vi "PhotonPoseEstimator_EstimatePnpDistanceTrigSolvePose.vi"(10 "CameraResult":T15={"Targets"=[], "PhotonMultiTargetPNPResult"={"PhotonPNPResult"={"IsPresent"=FALSE, "bestReprojErr"=0.0, "altReprojErr"=0.0, "ambiguity"=0.0, "Best"={"TRANSLATION3D"={"X"=0.0, "Y"=0.0, "Z"=0.0}, "ROTATION3D"={"Q_quaternion"={"R"=1.0, "V"=[0.0, 0.0, 0.0]}}, "XF"=FALSE}, "Alt"={"TRANSLATION3D"={"X"=0.0, "Y"=0.0, "Z"=0.0}, "ROTATION3D"={"Q_quaternion"={"R"=1.0, "V"=[0.0, 0.0, 0.0]}}, "XF"=FALSE}}, "FiducialIDsUsed"=[]}, "PhotonPipelineMetadata"={"CaptureTimestampMicros"=0, "PublishTimestampMicros"=0, "SequenceID"=0, "TimeSinceLastPong"=0}} {"PhotonMultiTargetPNPResult"."PhotonPNPResult"."Alt"."TRANSLATION3D"."Z" format="%14.3f"; "PhotonMultiTargetPNPResult"."PhotonPNPResult"."Alt"."TRANSLATION3D"."Y" format="%14.3f"; "PhotonMultiTargetPNPResult"."PhotonPNPResult"."Alt"."TRANSLATION3D"."X" format="%14.3f"; "PhotonMultiTargetPNPResult"."PhotonPNPResult"."Best"."TRANSLATION3D"."Z" format="%14.3f"; "PhotonMultiTargetPNPResult"."PhotonPNPResult"."Best"."TRANSLATION3D"."Y" format="%14.3f"; "PhotonMultiTargetPNPResult"."PhotonPNPResult"."Best"."TRANSLATION3D"."X" format="%14.3f"; "Targets"."AltCameraToTarget"."TRANSLATION3D"."Z" format="%14.3f"; "Targets"."AltCameraToTarget"."TRANSLATION3D"."Y" format="%14.3f"; "Targets"."AltCameraToTarget"."TRANSLATION3D"."X" format="%14.3f"; "Targets"."BestCameraToTarget"."TRANSLATION3D"."Z" format="%14.3f"; "Targets"."BestCameraToTarget"."TRANSLATION3D"."Y" format="%14.3f"; "Targets"."BestCameraToTarget"."TRANSLATION3D"."X" format="%14.3f"}, 11 "PhotoPoseEstimator":T1={"LastPose"={"Translation3d"={"X"=0.0, "Y"=0.0, "Z"=0.0}, "Rotation3d"={"Q_quaternion"={"R"=1.0, "V"=[0.0, 0.0, 0.0]}}}, "ReferencePose"={"Translation3d"={"X"=0.0, "Y"=0.0, "Z"=0.0}, "Rotation3d"={"Q_quaternion"={"R"=1.0, "V"=[0.0, 0.0, 0.0]}}}, "FieldTags"={"AprilTagMap"={}, "FieldLength"=0.0, "FieldWidth"=0.0, "OriginPosition "=enum."kBlueAllianceWallRightSide,", "OriginPose3d"={"Translation3d"={"X"=0.0, "Y"=0.0, "Z"=0.0}, "Rotation3d"={"Q_quaternion"={"R"=1.0, "V"=[0.0, 0.0, 0.0]}}}}, "PrimaryStratety"=enum."LOWEST_AMBIGUITY", "Camera"="", "RobotToCamera"={"TRANSLATION3D"={"X"=0.0, "Y"=0.0, "Z"=0.0}, "ROTATION3D"={"Q_quaternion"={"R"=1.0, "V"=[0.0, 0.0, 0.0]}}, "XF"=FALSE}, "ReportedErrors"=[], "HighestAmbiguity"=10.0, "MultiTagFallbackStrategy"=enum."LOWEST_AMBIGUITY", "PoseCacheTimeoutSec"=-1.0, "PhotonTargetModel"={"Vertices"=[], "IsPlaner"=FALSE, "IsSpherical"=FALSE}, "BaseNTName"="/photonvision"} {"PhotonTargetModel"."Vertices"."Z" format="%14.3f"; "PhotonTargetModel"."Vertices"."Y" format="%14.3f"; "PhotonTargetModel"."Vertices"."X" format="%14.3f"; "RobotToCamera"."TRANSLATION3D"."Z" format="%14.3f"; "RobotToCamera"."TRANSLATION3D"."Y" format="%14.3f"; "RobotToCamera"."TRANSLATION3D"."X" format="%14.3f"; "FieldTags"."OriginPose3d"."Translation3d"."Z" format="%14.3f"; "FieldTags"."OriginPose3d"."Translation3d"."Y" format="%14.3f"; "FieldTags"."OriginPose3d"."Translation3d"."X" format="%14.3f"; "ReferencePose"."Translation3d"."Z" format="%14.3f"; "ReferencePose"."Translation3d"."Y" format="%14.3f"; "ReferencePose"."Translation3d"."X" format="%14.3f"; "LastPose"."Translation3d"."Z" format="%14.3f"; "LastPose"."Translation3d"."Y" format="%14.3f"; "LastPose"."Translation3d"."X" format="%14.3f"}) -> (1 "Pos Found":bool, 3 "PhotonEstimatedRobotPose":T12={"EstimatedPose"={"Translation3d"={"X"=0.0, "Y"=0.0, "Z"=0.0}, "Rotation3d"={"Q_quaternion"={"R"=1.0, "V"=[0.0, 0.0, 0.0]}}}, "TimeStamp_Seconds"=0.0, "targetsUsed"=[], "Strategy"=enum."LOWEST_AMBIGUITY"} {"targetsUsed"."AltCameraToTarget"."TRANSLATION3D"."Z" format="%14.3f"; "targetsUsed"."AltCameraToTarget"."TRANSLATION3D"."Y" format="%14.3f"; "targetsUsed"."AltCameraToTarget"."TRANSLATION3D"."X" format="%14.3f"; "targetsUsed"."BestCameraToTarget"."TRANSLATION3D"."Z" format="%14.3f"; "targetsUsed"."BestCameraToTarget"."TRANSLATION3D"."Y" format="%14.3f"; "targetsUsed"."BestCameraToTarget"."TRANSLATION3D"."X" format="%14.3f"; "EstimatedPose"."Translation3d"."Z" format="%14.3f"; "EstimatedPose"."Translation3d"."Y" format="%14.3f"; "EstimatedPose"."Translation3d"."X" format="%14.3f"})   [LabVIEW 2019, in "PhotonVisionLib.lvlib"]
doc: "Return the estimated position of the robot by using distance data from best visible tag to compute a Pose. This runs on the RoboRIO in order to access the robot's yaw heading, and MUST have addHeadingData called every frame so heading data is up-to-date. \n\nYields a Pose2d in estimatedRobotPose (0 for z, roll, pitch)\n\nhttps://www.chiefdelphi.com/t/frc-6328-mechanical-advantage-2025-build-thread/477314/98\n\n\nInputs:\n -- PhotonPoseEstimator -- PhotonPoseEstimator -- data structure holding configuration.\n -- cameraResult -- PhotonPipelineResult -- A pipeline result from the camera.\n -- referencePose -- Pose3e -- last odometry calculated reference pose to check vector magnitude difference against.\n\nReturns:\n -- PhotonEstimatedRobotPose -- PhotonEstimatedRobotPose -- The with an estimated pose, timestamp, and targets used to create the estimate, or an empty optional if there's no targets.\n -- PosFound -- boolean -- TRUE if a position was found. If FALSE, no valid data was returned."
uses:
  PhotonVisionLib.lvlib
  TypeDef/PhotonPipelineResultType.ctl
  TypeDef/PhotonTrackedTargetType.ctl
  TypeDef/TargetCornerType.ctl
  <vilib>/Rock Robotics/WPI/ThirdParty/JAS_Junk/TrajLib/TypeDef/TRANSFORM3D.ctl
  <vilib>/Rock Robotics/WPI/ThirdParty/JAS_Junk/TrajLib/TypeDef/TRANSLATION3D.ctl
  <vilib>/Rock Robotics/WPI/ThirdParty/JAS_Junk/TrajLib/TypeDef/ROTATION3D.ctl
  <vilib>/Rock Robotics/WPI/ThirdParty/JAS_Junk/TrajLib/TypeDef/QUATERNION.ctl
  TypeDef/PhotonMultiTargetPNPResultType.ctl
  TypeDef/PhotonPNPResultType.ctl
  TypeDef/PhotonPipelineMetadataType.ctl
  TypeDef/PhotonEstimatedRobotPoseType.ctl
  <vilib>/Rock Robotics/WPI/ThirdParty/JAS_Junk/TrajLib/TypeDef/POSE3D.ctl
  Enum/PhotonPoseStrategy_ENUM.ctl
  TypeDef/PhotonPoseEstimatorType.ctl
  <vilib>/Rock Robotics/WPI/ThirdParty/JAS_Junk/TrajLib/TypeDef/AprilTagFieldLayout.ctl
  <vilib>/Rock Robotics/WPI/ThirdParty/JAS_Junk/TrajLib/TypeDef/AprilTag.ctl
  <vilib>/Rock Robotics/WPI/ThirdParty/JAS_Junk/TrajLib/Enum/AprilTagFieldLayoutOrignPosition_ENUM.ctl
  TypeDef/PhotonTargetModel.ctl
  <vilib>/Rock Robotics/WPI/ThirdParty/JAS_Junk/TrajLib/VI/Quaternion_New.vi
  <vilib>/Rock Robotics/WPI/ThirdParty/JAS_Junk/TrajLib/Conv_Deg_Radians.vi
  <vilib>/Rock Robotics/WPI/ThirdParty/JAS_Junk/TrajLib/VI/Rotation3d_ToRotation2d.vi
  <vilib>/Rock Robotics/WPI/ThirdParty/JAS_Junk/TrajLib/Transform2d_Create_TransRot.vi
  <vilib>/Rock Robotics/WPI/ThirdParty/JAS_Junk/TrajLib/VI/Translation3d_Create.vi
  <vilib>/Rock Robotics/WPI/ThirdParty/JAS_Junk/TrajLib/VI/Rotation3d_GetQuaterion.vi
  <vilib>/Rock Robotics/WPI/ThirdParty/JAS_Junk/TrajLib/VI/Quaternion_Times.vi
  <vilib>/Rock Robotics/WPI/ThirdParty/JAS_Junk/TrajLib/VI/Quaternion_Inverse.vi
  <vilib>/Rock Robotics/WPI/ThirdParty/JAS_Junk/TrajLib/VI/Quaternion_Get_All.vi
  <vilib>/Rock Robotics/WPI/ThirdParty/JAS_Junk/TrajLib/Translation2d_Create.vi
  <vilib>/Rock Robotics/WPI/ThirdParty/JAS_Junk/TrajLib/VI/Pose3d_getTranslation3d.vi
  <vilib>/Rock Robotics/WPI/ThirdParty/JAS_Junk/TrajLib/VI/Pose3d_getRotation3d.vi
  <vilib>/Rock Robotics/WPI/ThirdParty/JAS_Junk/TrajLib/VI/Pose3d_New_Trans3dRot3d.vi
  <vilib>/Rock Robotics/WPI/ThirdParty/JAS_Junk/TrajLib/Pose2d_getXYAngle.vi
  <vilib>/Rock Robotics/WPI/ThirdParty/JAS_Junk/TrajLib/Rotation2d_Interpolate.vi
  <vilib>/Rock Robotics/WPI/ThirdParty/JAS_Junk/TrajLib/VI/AprilTag_GetAll.vi
  <vilib>/Rock Robotics/WPI/ThirdParty/JAS_Junk/TrajLib/VI/Pose3d_RelativeTo.vi
  <vilib>/Rock Robotics/WPI/ThirdParty/JAS_Junk/TrajLib/VI/Rotation3d_Create_AxisAngle.vi
  <vilib>/Rock Robotics/WPI/ThirdParty/JAS_Junk/TrajLib/VI/Pose3d_New.vi
  <vilib>/Rock Robotics/WPI/ThirdParty/JAS_Junk/TrajLib/Rotation2d_CreateAngle.vi
  <vilib>/Rock Robotics/WPI/ThirdParty/JAS_Junk/TrajLib/VI/Rotation3d_GetXYZ.vi
  <vilib>/Rock Robotics/WPI/ThirdParty/JAS_Junk/TrajLib/Rotation2d_Plus.vi
  <vilib>/Rock Robotics/WPI/ThirdParty/JAS_Junk/TrajLib/Rotation2d_Minus.vi
  <vilib>/Rock Robotics/WPI/ThirdParty/JAS_Junk/TrajLib/MathUtil_Clamp.vi
  <vilib>/Rock Robotics/WPI/ThirdParty/JAS_Junk/TrajLib/Rotation2d_Times.vi
  <vilib>/Rock Robotics/WPI/ThirdParty/JAS_Junk/TrajLib/VI/Transform3d_Create_Pose3dPose3d.vi
  <vilib>/Rock Robotics/WPI/ThirdParty/JAS_Junk/TrajLib/VI/Rotation3d_Create_Default.vi
  <vilib>/Rock Robotics/WPI/ThirdParty/JAS_Junk/TrajLib/VI/Vector_Norm.vi
  <vilib>/Rock Robotics/WPI/ThirdParty/JAS_Junk/TrajLib/VecBuilder_ArrayBy1Fill.vi
  <vilib>/Rock Robotics/WPI/ThirdParty/JAS_Junk/TrajLib/Rotation2d_RotateBy.vi
  <vilib>/Rock Robotics/WPI/ThirdParty/JAS_Junk/TrajLib/Rotation2d_UnaryMinus.vi
  <vilib>/Rock Robotics/WPI/ThirdParty/JAS_Junk/TrajLib/VI/Transform3d_Create_Trans3dRot3d.vi
  <vilib>/Rock Robotics/WPI/ThirdParty/JAS_Junk/TrajLib/VI/Translation3d_Minus.vi
  <vilib>/Rock Robotics/WPI/ThirdParty/JAS_Junk/TrajLib/VI/Rotation3d_UnaryMinus.vi
  <vilib>/Rock Robotics/WPI/ThirdParty/JAS_Junk/TrajLib/VI/Rotation3d_Minus.vi
  <vilib>/Rock Robotics/WPI/ThirdParty/JAS_Junk/TrajLib/VI/Quaternion_New_Default.vi
  <vilib>/Rock Robotics/WPI/ThirdParty/JAS_Junk/TrajLib/MatBuilder_Create.vi
  <vilib>/Rock Robotics/WPI/ThirdParty/JAS_Junk/TrajLib/Rotation2d_CreateXY.vi
  <vilib>/Rock Robotics/WPI/ThirdParty/JAS_Junk/TrajLib/VI/Rotation3d_Create_Quaternion.vi
  <vilib>/Rock Robotics/WPI/ThirdParty/JAS_Junk/TrajLib/VI/Rotation3d_RotateBy.vi
  <vilib>/Rock Robotics/WPI/ThirdParty/JAS_Junk/TrajLib/Util_CalcDist.vi
  <vilib>/Rock Robotics/WPI/ThirdParty/JAS_Junk/TrajLib/VI/Quaternion_Normalize.vi
  PhotonVision_Globals.vi
  <vilib>/gmath/interp.llb/Search Ordered Table.vi
  <vilib>/Rock Robotics/WPI/ThirdParty/JAS_Junk/TrajLib/Trajectory_Library.lvlib
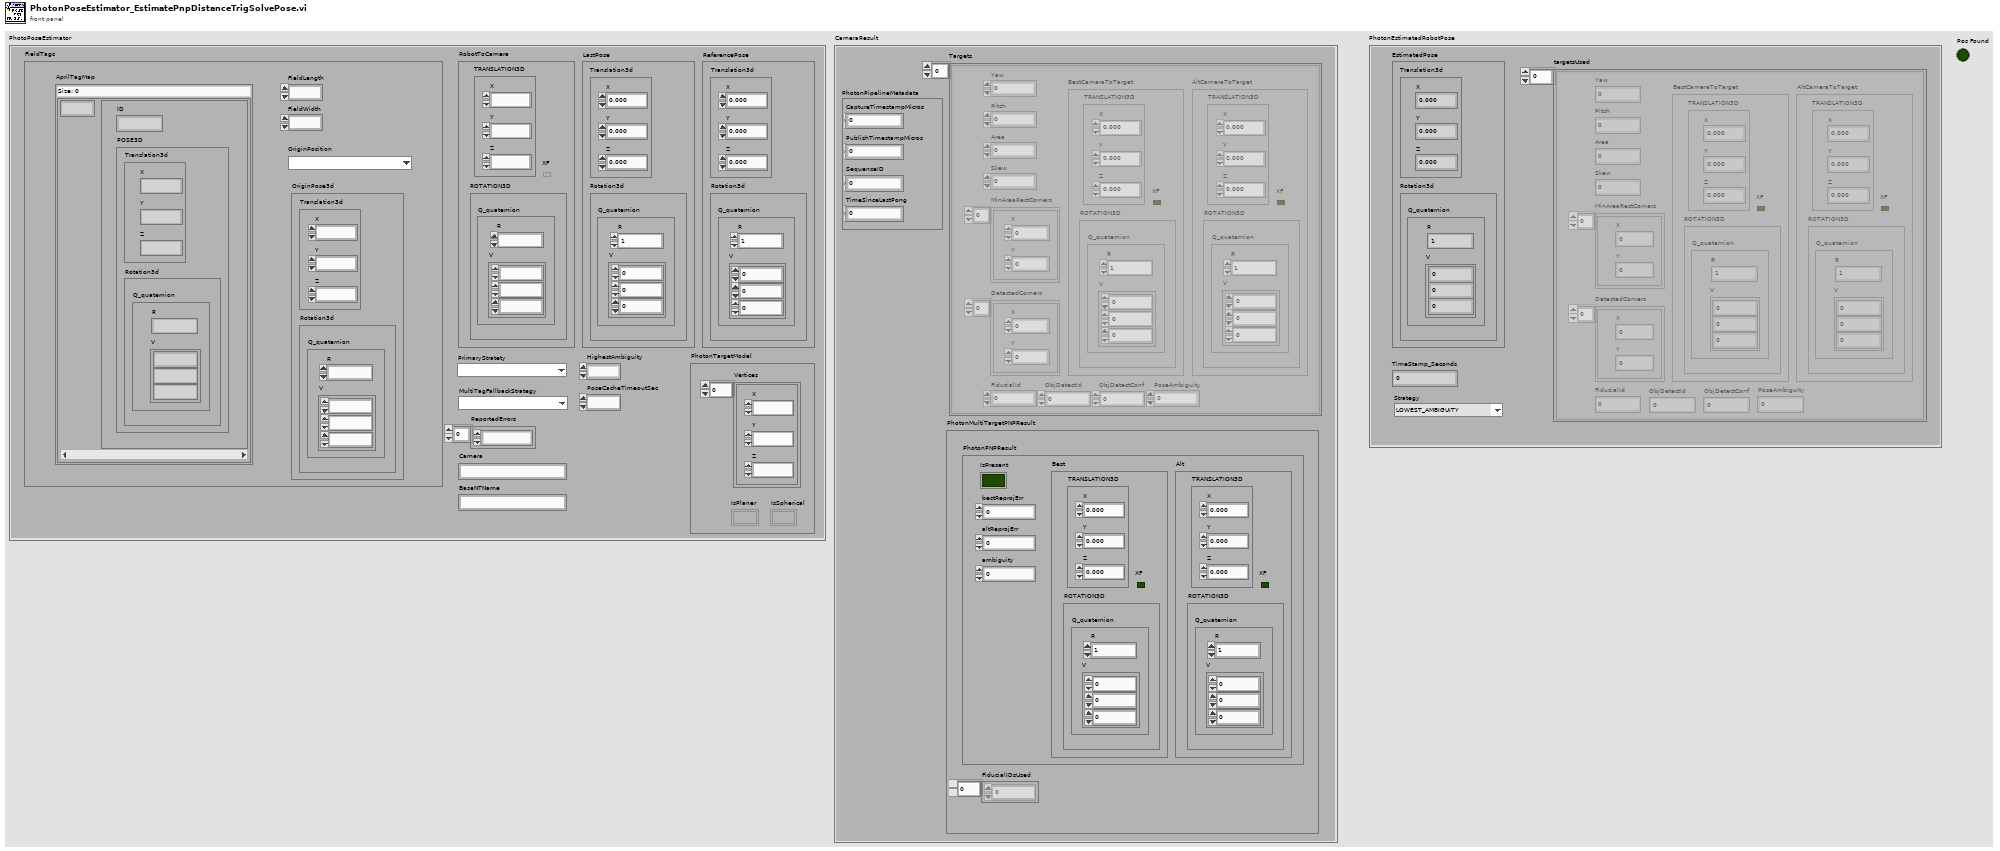
[diagram p1: front panel]
types:
  T1 = typedef "PhotonVisionLib.lvlib/PhotonPoseEstimatorType.ctl" = cluster{"LastPose":T2, "ReferencePose":T2, "FieldTags":T6, "PrimaryStratety":T9, "Camera":string, "RobotToCamera":T10, "ReportedErrors":dbl[], "HighestAmbiguity":dbl, "MultiTagFallbackStrategy":T9, "PoseCacheTimeoutSec":dbl, "PhotonTargetModel":T11, "BaseNTName":string}
  T2 = typedef "Trajectory_Library.lvlib/POSE3D.ctl" = cluster{"Translation3d":T3, "Rotation3d":T4}
  T3 = typedef "Trajectory_Library.lvlib/TRANSLATION3D.ctl" = cluster{"X":dbl, "Y":dbl, "Z":dbl}
  T4 = typedef "Trajectory_Library.lvlib/ROTATION3D.ctl" = cluster{"Q_quaternion":T5}
  T5 = typedef "Trajectory_Library.lvlib/QUATERNION.ctl" = cluster{"R":dbl, "V":dbl[]}
  T6 = typedef "Trajectory_Library.lvlib/AprilTagFieldLayout.ctl" = cluster{"AprilTagMap":map{i32, T7}, "FieldLength":dbl, "FieldWidth":dbl, "OriginPosition ":T8, "OriginPose3d":T2}
  T7 = typedef "Trajectory_Library.lvlib/AprilTag.ctl" = cluster{"ID":i32, "POSE3D":T2}
  T8 = typedef "Trajectory_Library.lvlib/AprilTagFieldLayoutOrignPosition_ENUM.ctl" = enum16{"kBlueAllianceWallRightSide,", "kRedAllianceWallRightSide,"}
  T9 = typedef "PhotonVisionLib.lvlib/PhotonPoseStrategy_ENUM.ctl" = enum16{"LOWEST_AMBIGUITY", "CLOSEST_TO_CAMERA_HEIGHT", "CLOSEST_TO_REFERENCE_POSE", "CLOSEST_TO_LAST_POSE", "AVERAGE_BEST_TARGETS", "MULTI_TAG_PNP_ON_COPROCESSOR", "MULTI_TAG_PNP_ON_RIO", "PNP_DISTANCE_TRIG_SOLVE", "CONSTRAINED_SOLVEPNP"}
  T10 = typedef "Trajectory_Library.lvlib/TRANSFORM3D.ctl" = cluster{"TRANSLATION3D":T3, "ROTATION3D":T4, "XF":bool}
  T11 = typedef "PhotonVisionLib.lvlib/PhotonTargetModel.ctl" = cluster{"Vertices":T3[], "IsPlaner":bool, "IsSpherical":bool}
  T12 = typedef "PhotonVisionLib.lvlib/PhotonEstimatedRobotPoseType.ctl" = cluster{"EstimatedPose":T2, "TimeStamp_Seconds":dbl, "targetsUsed":T13[], "Strategy":T9}
  T13 = typedef "PhotonVisionLib.lvlib/PhotonTrackedTargetType.ctl" = cluster{"Yaw":dbl, "Pitch":dbl, "Area":dbl, "Skew":dbl, "MinAreaRectCorners":T14[], "BestCameraToTarget":T10, "FiducialId":i32, "AltCameraToTarget":T10, "PoseAmbiguity":dbl, "DetectedCorners":T14[], "ObjDetectId":i32, "ObjDetectConf":sgl}
  T14 = typedef "PhotonVisionLib.lvlib/TargetCornerType.ctl" = cluster{"X":dbl, "Y":dbl}
  T15 = typedef "PhotonVisionLib.lvlib/PhotonPipelineResultType.ctl" = cluster{"Targets":T13[], "PhotonMultiTargetPNPResult":T16, "PhotonPipelineMetadata":T18}
  T16 = typedef "PhotonVisionLib.lvlib/PhotonMultiTargetPNPResultType.ctl" = cluster{"PhotonPNPResult":T17, "FiducialIDsUsed":i16[]}
  T17 = typedef "PhotonVisionLib.lvlib/PhotonPNPResultType.ctl" = cluster{"IsPresent":bool, "bestReprojErr":dbl, "altReprojErr":dbl, "ambiguity":dbl, "Best":T10, "Alt":T10}
  T18 = typedef "PhotonVisionLib.lvlib/PhotonPipelineMetadataType.ctl" = cluster{"CaptureTimestampMicros":i64, "PublishTimestampMicros":i64, "SequenceID":i64, "TimeSinceLastPong":i64}
  T19 = typedef "Trajectory_Library.lvlib/TIME_INTERPOLATABLE_ROTATION2D.ctl" = cluster{"TimeStamps":dbl[], "RotationValues":T20[], "Min_TimeStamp":dbl, "Max_TimeStamp":dbl, "ItemCount":i32, "MaxBufferTime":dbl}
  T20 = typedef "Trajectory_Library.lvlib/ROTATION2D.ctl" = cluster{"VALUE":dbl, "COS":dbl, "SIN":dbl}
  T21 = typedef "Trajectory_Library.lvlib/POSE2D.ctl" = cluster{"TRANSLATION":T22, "ROTATION":T20}
  T22 = typedef "Trajectory_Library.lvlib/TRANSLATION2D.ctl" = cluster{"X":dbl, "Y":dbl}
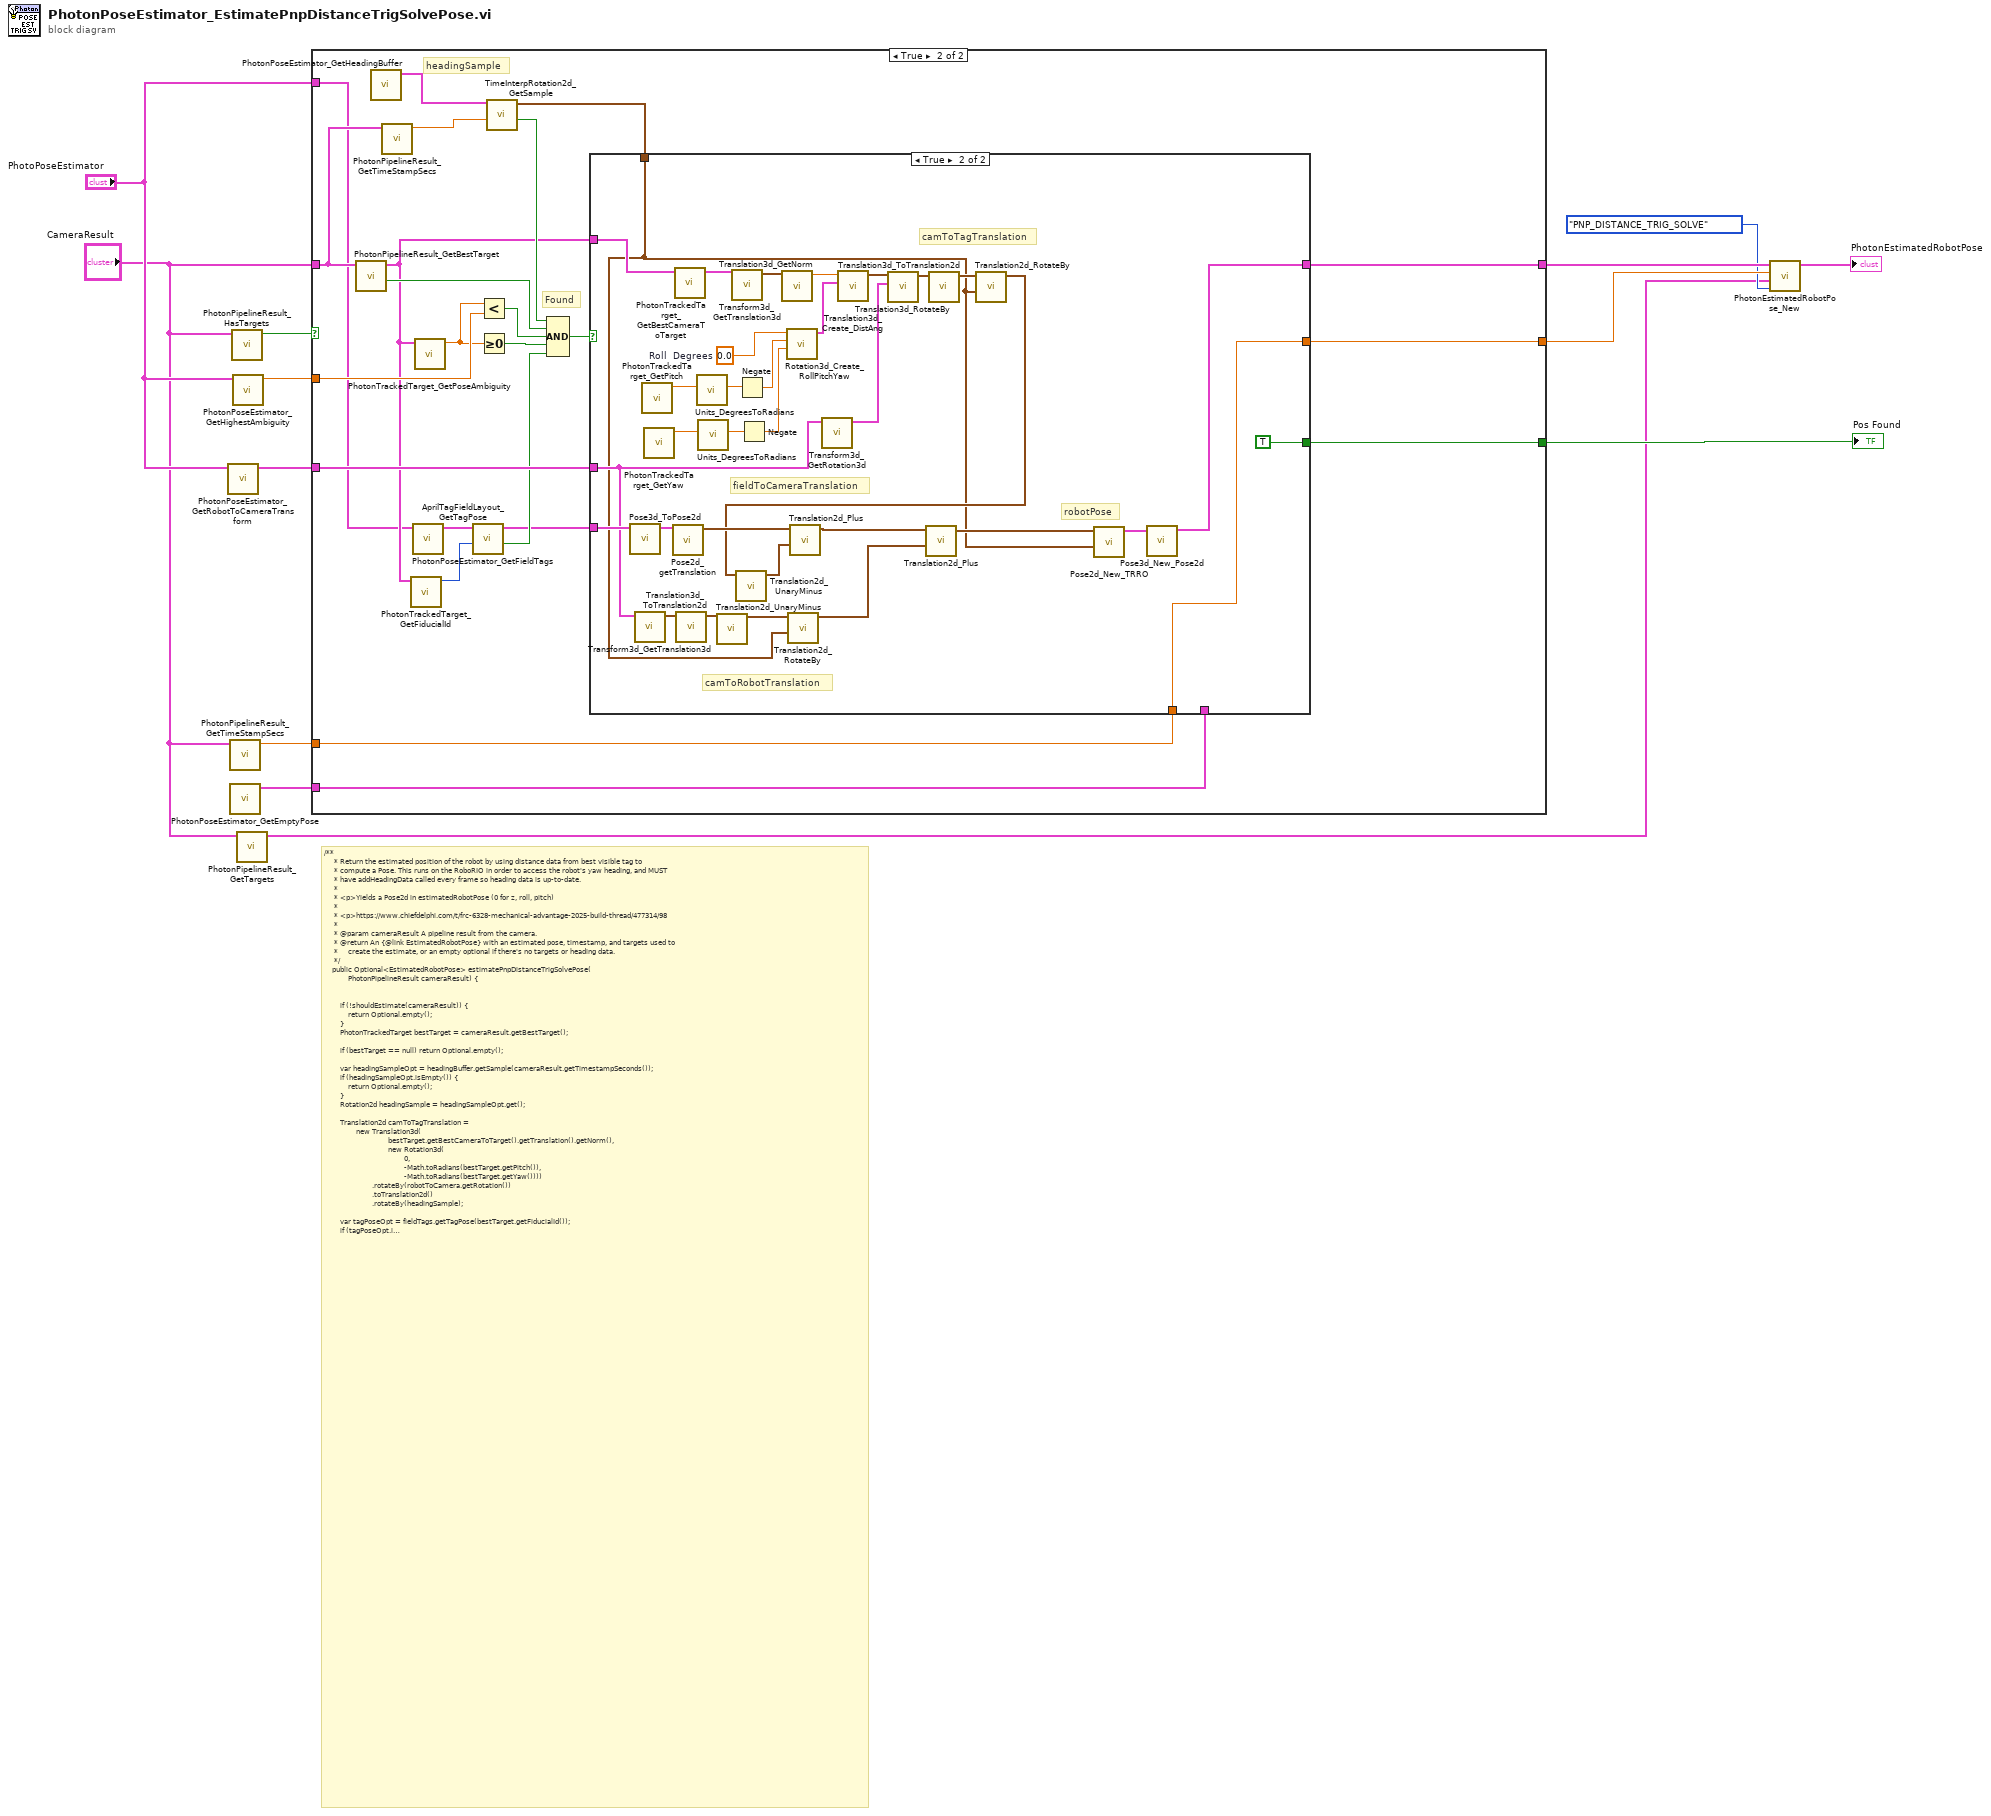
[diagram p0: block diagram]
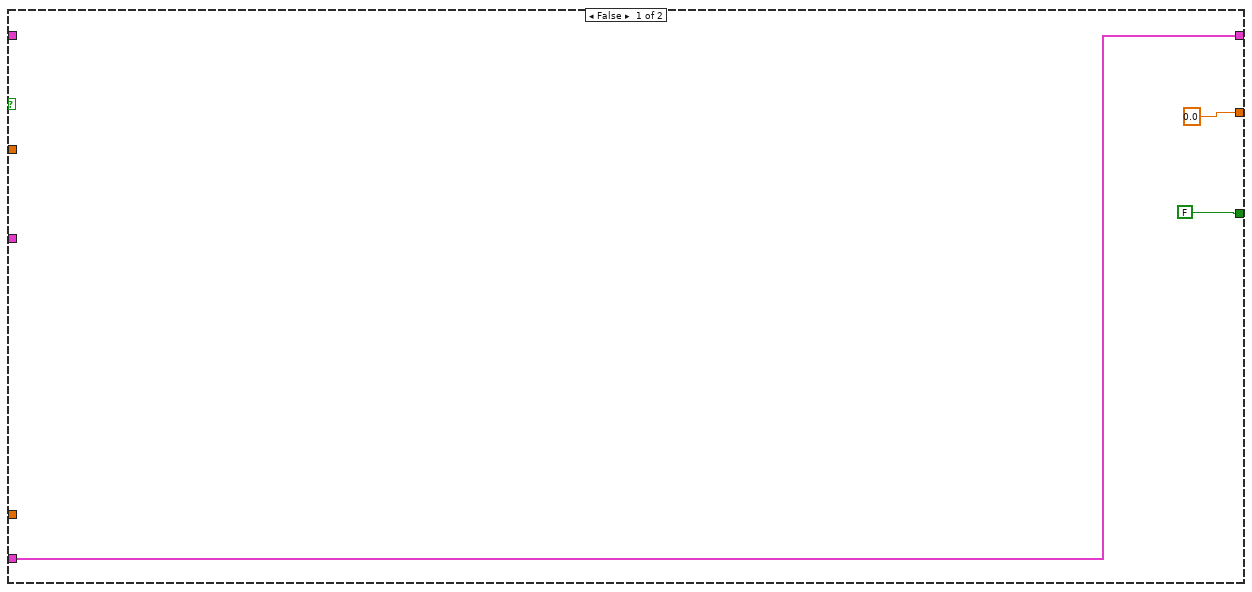
[diagram p2: hidden frame]
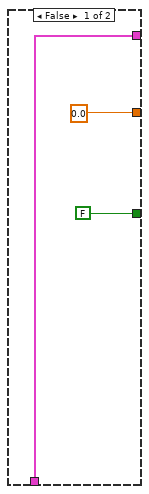
[diagram p3: hidden frame]
diagram:
  # "/**\n     * Return the estimated position of the robot by using distance data from best visible tag to\n     * compute a Pose. This runs on the RoboRIO in order to access the robot's yaw heading, and MUST\n     * have addHeadingData called every frame so heading data is up-to-date.\n     *\n     * <p>Yields a Pose2d in estimatedRobotPose (0 for z, roll, pitch)\n     *\n     * <p>https://www.chiefdelphi.com/t/frc-6328-mechanical-advantage-2025-build-thread/477314/98\n     *\n     * @param cameraResult A pipeline result from the camera.\n     * @return An {@link EstimatedRobotPose} with an estimated pose, timestamp, and targets used to\n     *     create the estimate, or an empty optional if there's no targets or heading data.\n     */\n    public Optional<EstimatedRobotPose> estimatePnpDistanceTrigSolvePose(\n            PhotonPipelineResult cameraResult) {\n\n\n        if (!shouldEstimate(cameraResult)) {\n            return Optional.empty();\n        }\n        PhotonTrackedTarget bestTarget = cameraResult.getBestTarget();\n\n        if (bestTarget == null) return Optional.empty();\n\n        var headingSampleOpt = headingBuffer.getSample(cameraResult.getTimestampSeconds());\n        if (headingSampleOpt.isEmpty()) {\n            return Optional.empty();\n        }\n        Rotation2d headingSample = headingSampleOpt.get();\n\n        Translation2d camToTagTranslation =\n                new Translation3d(\n                                bestTarget.getBestCameraToTarget().getTranslation().getNorm(),\n                                new Rotation3d(\n                                        0,\n                                        -Math.toRadians(bestTarget.getPitch()),\n                                        -Math.toRadians(bestTarget.getYaw())))\n                        .rotateBy(robotToCamera.getRotation())\n                        .toTranslation2d()\n                        .rotateBy(headingSample);\n\n        var tagPoseOpt = fieldTags.getTagPose(bestTarget.getFiducialId());\n        if (tagPoseOpt.isEmpty()) {\n            return Optional.empty();\n        }\n        var tagPose2d = tagPoseOpt.get().toPose2d();\n\n        Translation2d fieldToCameraTranslation =\n                tagPose2d.getTranslation().plus(camToTagTranslation.unaryMinus());\n\n        Translation2d camToRobotTranslation =\n                robotToCamera.getTranslation().toTranslation2d().unaryMinus().rotateBy(headingSample);\n\n        Pose2d robotPose =\n                new Pose2d(fieldToCameraTranslation.plus(camToRobotTranslation), headingSample);\n\n        return Optional.of(\n                new EstimatedRobotPose(\n                        new Pose3d(robotPose),\n                        cameraResult.getTimestampSeconds(),\n                        cameraResult.getTargets(),\n                        PoseStrategy.PNP_DISTANCE_TRIG_SOLVE));\n    }"
  n1 = call "PhotonPoseEstimator_GetRobotToCameraTransform.vi"("PhotonPoseEstimator"="PhotoPoseEstimator") -> ("RobotToCamera"=w10:T10)  [unwired: 10 in]
  n2 = call "PhotonPipelineResult_GetTimeStampSecs.vi"("PhotonPipelineResult"="CameraResult") -> ("TimeStampSec"=w11:dbl)  [unwired: 10 in]
  n3 = call "PhotonPoseEstimator_GetEmptyPose.vi"() -> ("EmptyPose"=w9:T2)  [unwired: 11 in]
  n4 = call "PhotonPipelineResult_HasTargets.vi"("PhotonPipelineResult"="CameraResult") -> ("HasTargets"=w13:bool)  [unwired: 10 in]
  n5 = call "PhotonPoseEstimator_GetHighestAmbiguity.vi"("PhotonPoseEstimator"="PhotoPoseEstimator") -> ("HighestAmbiguity"=w7:dbl)  [unwired: 10 in]
  n6 = call "PhotonPipelineResult_GetTargets.vi"("PhotonPipelineResult"="CameraResult") -> ("Targets"=w1:T13[])  [unwired: 10 in]
  n7 = case shown="True" w13 {
    tunnel: "CameraResult" -> [_ w33]
    tunnel: [FALSE ("Found") w39] -> w12
    tunnel: "PhotoPoseEstimator" -> [_ w22]
    tunnel: w11 -> [_ w19]
    tunnel: w10 -> [_ w29]
    tunnel: w9 -> [w15 w21]
    tunnel: w7 -> [_ w38]
    tunnel: [0.0 ("TimeStamp_Seconds") w18] -> w6
    tunnel: [w15 w20] -> w5
    frame False {
    }
    frame True {
      # "headingSample"
      # "Found"
      n8 = call "PhotonPipelineResult_GetBestTarget.vi"("PhotonPipelineResult"=w33) -> ("TargetFound"=w30:bool, "PhotonTrackedTarget"=w27:T13)  [unwired: 9 in]
      n9 = call "PhotonPoseEstimator_GetHeadingBuffer.vi"() -> ("PoseEstimatorHeadingBuffer"=w17:T19)  [unwired: 11 in]
      n10 = call "PhotonPipelineResult_GetTimeStampSecs.vi"("PhotonPipelineResult"=w33) -> ("TimeStampSec"=w32:dbl)  [unwired: 10 in]
      n11 = call "PhotonTrackedTarget_GetFiducialId.vi"("TrackedTarget"=w27) -> ("Fiducial Id"=w25:i32)  [unwired: 10 in]
      n12 = call "PhotonPoseEstimator_GetFieldTags.vi"("PhotonPoseEstimator"=w22) -> ("AprilTagFieldLayout"=w26:T6)  [unwired: 10 in]
      n13 = call "PhotonTrackedTarget_GetPoseAmbiguity.vi"("TrackedTarget"=w27) -> ("Pose Ambiguity"=w35:dbl)  [unwired: 10 in]
      n14 = call <vilib>:"AprilTagFieldLayout_GetTagPose.vi"("TagId"=w25, "AprilTagFieldLayout"=w26) -> ("Found"=w24:bool, "TagPose3d"=w23:T2)  [unwired: 8 in]
      n15 = Less?(x=w35, y=w38) -> (x < y?=w34:bool)
      n16 = Greater Or Equal To 0?(x=w35) -> (x >= 0?=w37:bool)
      n17 = call <vilib>:"TimeInterpRotation2d_GetSample.vi"("TimeStamp"=w32, "TimeInterpRotation"=w17) -> ("IsPresent"=w31:bool, "OutputRotation"=w28:T20)  [unwired: 8 in]
      n18 = Compound Arithmetic op=AND(w31, w30, w34, w37, w24) -> (w36:bool)
      n19 = case shown="True" w36 {
        tunnel: [FALSE TRUE] -> w39
        tunnel: w27 -> [_ w59]
        tunnel: w29 -> [_ w53]
        tunnel: w28 -> [_ w46]
        tunnel: w23 -> [_ w58]
        tunnel: [w41 w44] -> w20
        tunnel: w21 -> [w41 _]
        tunnel: w19 -> [_ w43]
        tunnel: [0.0 ("TimeStamp_Seconds") w43] -> w18
        frame False {
        }
        frame True {
          w74 = 0.0  # Roll  Degrees
          # "robotPose"
          # "camToRobotTranslation"
          # "fieldToCameraTranslation"
          # "camToTagTranslation"
          n20 = call <vilib>:"Pose3d_ToPose2d.vi"("in Pose3d"=w58) -> ("out Pose2d"=w57:T21)  [unwired: 10 in]
          n21 = call <vilib>:"Transform3d_GetTranslation3d.vi"("in Transform3d"=w53) -> ("Translation3d"=w52:T3)  [unwired: 10 in]
          n22 = call "PhotonTrackedTarget_GetPitch.vi"() -> ("Pitch"=w73:dbl)  [unwired: 11 in]
          n23 = call "PhotonTrackedTarget_GetYaw.vi"() -> ("Yaw"=w72:dbl)  [unwired: 11 in]
          n24 = call <vilib>:"Pose2d_getTranslation.vi"("in POSE"=w57) -> ("outTRANSLATION"=w56:T22)  [unwired: 10 in]
          n25 = call "PhotonTrackedTarget_GetBestCameraToTarget.vi"("TrackedTarget"=w59) -> ("BestCameraToTarget"=w67:T10)  [unwired: 9 in, 1 out]
          n26 = call <vilib>:"Translation3d_ToTranslation2d.vi"("In Translation3d"=w52) -> ("Translation2d"=w51:T22)  [unwired: 10 in]
          n27 = call <vilib>:"Units_DegreesToRadians.vi"("Degrees"=w73) -> ("Radians"=w71:dbl)  [unwired: 10 in]
          n28 = call <vilib>:"Units_DegreesToRadians.vi"("Degrees"=w72) -> ("Radians"=w70:dbl)  [unwired: 10 in]
          n29 = call <vilib>:"Translation2d_UnaryMinus.vi"("In Translation"=w51) -> ("Out Translation"=w50:T22)  [unwired: 10 in]
          n30 = call <vilib>:"Transform3d_GetTranslation3d.vi"("in Transform3d"=w67) -> ("Translation3d"=w66:T3)  [unwired: 10 in]
          n31 = Negate(x=w71) -> (-x=w68:dbl)
          n32 = Negate(x=w70) -> (-x=w69:dbl)
          n33 = call <vilib>:"Translation3d_GetNorm.vi"("In Translation3d"=w66) -> ("Norm"=w65:dbl)  [unwired: 10 in]
          n34 = call <vilib>:"Rotation3d_Create_RollPitchYaw.vi"("Yaw"=w69, "Pitch"=w68, "Roll"=w74) -> ("Rotation3d"=w64:T4)  [unwired: 8 in]
          n35 = call <vilib>:"Translation2d_RotateBy.vi"("other Rotation"=w46, "In Translation"=w50) -> ("Out Translation"=w48:T22)  [unwired: 9 in]
          n36 = call <vilib>:"Transform3d_GetRotation3d.vi"("in Transform3d"=w53) -> ("Rotation3d"=w60:T4)  [unwired: 10 in]
          n37 = call <vilib>:"Translation3d_Create_DistAng.vi"("Angle_Rotation3d"=w64, "Distance"=w65) -> ("TRANSLATION3D"=w63:T3)  [unwired: 9 in]
          n38 = call <vilib>:"Translation3d_RotateBy.vi"("other Rot3d"=w60, "in Translation3D"=w63) -> ("out Translation3d"=w62:T3)  [unwired: 9 in]
          n39 = call <vilib>:"Translation3d_ToTranslation2d.vi"("In Translation3d"=w62) -> ("Translation2d"=w61:T22)  [unwired: 10 in]
          n40 = call <vilib>:"Translation2d_RotateBy.vi"("other Rotation"=w46, "In Translation"=w61) -> ("Out Translation"=w54:T22)  [unwired: 9 in]
          n41 = call <vilib>:"Translation2d_UnaryMinus.vi"("In Translation"=w54) -> ("Out Translation"=w55:T22)  [unwired: 10 in]
          n42 = call <vilib>:"Translation2d_Plus.vi"("other Translation"=w55, "In Translation"=w56) -> ("Out Translation"=w49:T22)  [unwired: 9 in]
          n43 = call <vilib>:"Translation2d_Plus.vi"("other Translation"=w48, "In Translation"=w49) -> ("Out Translation"=w47:T22)  [unwired: 9 in]
          n44 = call <vilib>:"Pose2d_New_TRRO.vi"("ROTATION"=w46, "TRANSLATION"=w47) -> ("outPOSE"=w45:T21)  [unwired: 9 in]
          n45 = call <vilib>:"Pose3d_New_Pose2d.vi"("in POSE2D"=w45) -> ("out Pose3d"=w44:T2)  [unwired: 10 in]
        }
      }
    }
  }
  "Pos Found" <- w12
  n46 = call "PhotonEstimatedRobotPose_New.vi"("Strategy"=PhotonPoseStrategy_ENUM."PNP_DISTANCE_TRIG_SOLVE", "targetsUsed"=w1, "TimeStamp_Seconds"=w6, "EstimatedPose"=w5) -> ("PhotonEstimatedRobotPose"=→"PhotonEstimatedRobotPose":T12)  [unwired: 7 in]
